vi "Brace_get_filename.vi"(11 "Directory":path) -> (0 "error out":errorcluster, 1 "Filename":string, 3 "refnum out":refnum<file>)   [LabVIEW 2018]
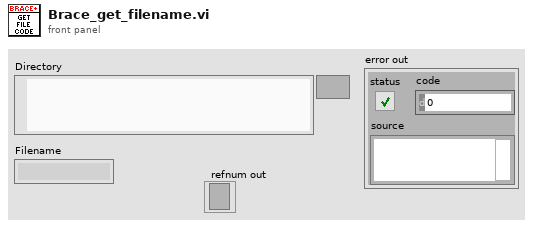
[diagram p1: front panel]
types:
  T1 = enum16{"open", "replace", "create", "open or create", "replace or create", "replace or create with confirmation"}
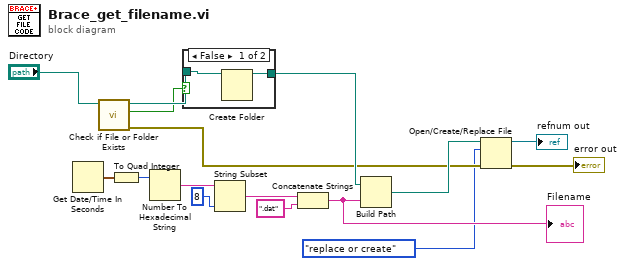
[diagram p0: block diagram]
diagram:
  n1 = Get Date/Time In Seconds() -> (seconds since 1Jan1904=w14:timestamp)
  n2 = call <vilib>:"Check if File or Folder Exists.vi"("path"="Directory") -> ("error out"=w4:errorcluster, "file or folder exists?"=w8:bool, "dup path"=w9:path)  [unwired: 8 in]
  n3 = To Quad Integer(1:w14) -> (0:w15:i64)
  n4 = Number To Hexadecimal String(2:w15) -> (0:w16:string)  [unwired: 1 in]
  n5 = case shown="False" w8 {
    tunnel: w9 -> [w18 w19]
    tunnel: [w17 w19] -> w6
    frame False {
      n6 = Create Folder(path (use dialog)=w18) -> (created path=w17:path)  [unwired: 2 in, 2 out]
    }
    frame True {
    }
  }
  n7 = String Subset(string=w16, length (rest)=i16 8 ("Elapsed Time (ms)")) -> (substring=w10:string)  [unwired: 1 in]
  n8 = Concatenate Strings(w10, ".dat" ("string")) -> (w12:string)
  "Filename" <- w12
  n9 = Build Path(base path=w6, name or relative path=w12) -> (appended path=w5:path)
  n10 = Open/Create/Replace File(file path (use dialog)=w5, error in=w4, operation (0:open)=T1."replace or create") -> (refnum out=→"refnum out":refnum<file>, error out=→"error out":errorcluster)  [unwired: 3 in, 1 out]
